vi "moveStageREL_z.vi"(4 "Radio Buttons":enum32{"Coarse (mm) ", "Fine (um) "}(radio)=enum."Fine (um) ", 5 "increment":dbl, 6 "initPos (mm)":dbl, 7 "stage lim (mm)":dbl, 8 "axisIdx":i32, 9 "System no.":i32=1 min=1 max=4 step=1, 10 "stageInit":i16) -> (2 "finPos":dbl)   [LabVIEW 2015]
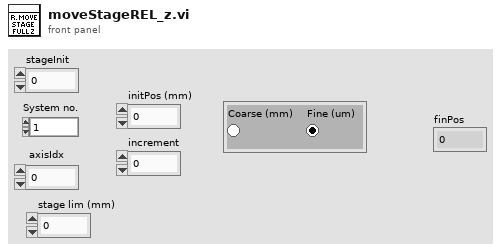
[diagram p1: front panel]
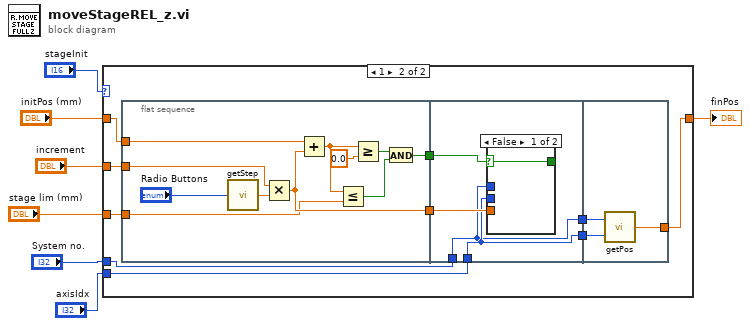
[diagram p0: block diagram]
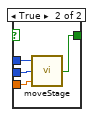
[diagram p3: hidden frame]
diagram:
  n1 = case shown="1" "stageInit" {
    tunnel: [w8 w17] -> w7
    tunnel: "initPos (mm)" -> [w8 w14]
    tunnel: "System no." -> [_ w16]
    tunnel: "axisIdx" -> [_ w15]
    tunnel: "increment" -> [_ w13]
    tunnel: "stage lim (mm)" -> [_ w10]
    frame 0, Default {
    }
    frame 1 {
      n2 = flat-sequence {
        tunnel: [w28] -> w18
        tunnel: w14 -> [w26]
        tunnel: w13 -> [w25]
        tunnel: w10 -> [w24]
        tunnel: [w21] -> w9
        tunnel: w18 -> [w33]
        tunnel: w16 -> [w31]
        tunnel: w15 -> [w32]
        tunnel: [w32] -> w12
        tunnel: [w31] -> w11
        tunnel: w9 -> [w30]
        tunnel: [w41] -> w17
        tunnel: w12 -> [w40]
        tunnel: w11 -> [w39]
        frame #0 {
          n3 = call "getStep.vi"("Radio Buttons"="Radio Buttons") -> ("step"=w29:dbl)
          n4 = Multiply(x=w25, y=w29) -> (x*y=w28:dbl)
          n5 = Add(x=w26, y=w28) -> (x+y=w20:dbl)
          n6 = Less Or Equal?(x=w20, y=w24) -> (x <= y?=w22:bool)
          n7 = Greater Or Equal?(x=w20, y=0.0 ("x")) -> (x >= y?=w23:bool)
          n8 = And(x=w23, y=w22) -> (x .and. y?=w21:bool)
        }
        frame #1 {
          n9 = case shown="False" w30 {
            selector: w30 -> [w34 _]
            tunnel: [w34 w38] -> _
            tunnel: w33 -> [_ w37]
            tunnel: w31 -> [_ w36]
            tunnel: w32 -> [_ w35]
            frame False {
            }
            frame True {
              n10 = call "moveStage.vi"("inc (mm)"=w37, "axisIdx"=w35, "System no."=w36) -> ("Stopped"=w38:bool)
            }
          }
        }
        frame #2 {
          n11 = call "getPos.vi"("axisIdx"=w40, "System no."=w39) -> ("stagePos"=w41:dbl)
        }
      }
    }
  }
  "finPos" <- w7
